vi "_Engine.vi"(6 "Enum":T1, 7 "Module Name":string, 8 "Error in":errorcluster caption="Error in (no error)", 11 "Message":string) -> (0 "Error out":errorcluster, 2 "Array":string[](array[string]), 3 "Message Event":refnum<user-event>)   [LabVIEW 2017, in "_csmlite.lvlib"]
uses:
  _csmlite.lvlib
  _action.ctl
  _Shared/CSM Shared.lvlib
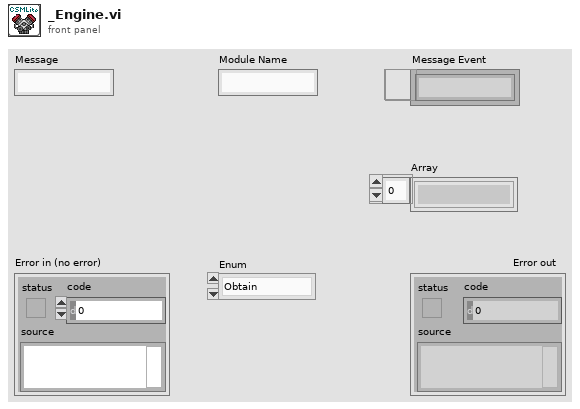
[diagram p1: front panel]
types:
  T1 = typedef "_csmlite.lvlib/_action.ctl" = enum16{"Obtain", "Destroy", "Broadcast", "Post", "List"}
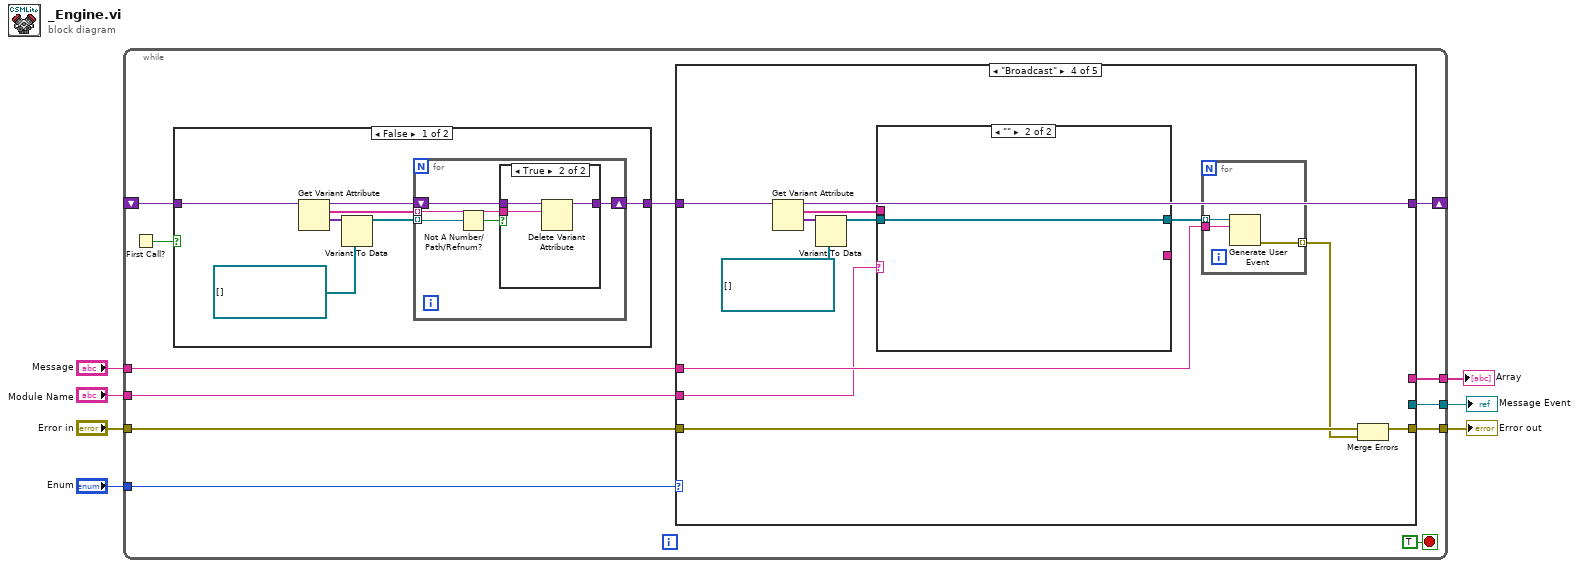
[diagram p0: block diagram]
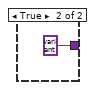
[diagram p3: hidden frame]
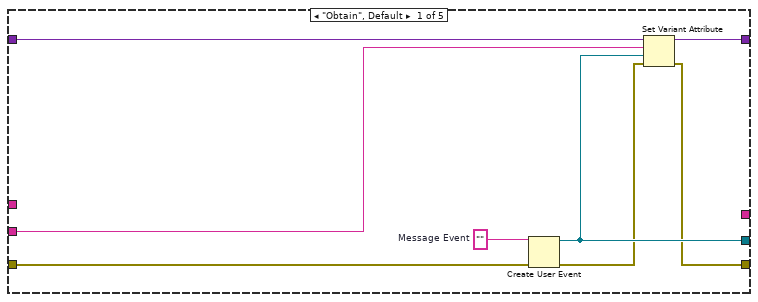
[diagram p4: hidden frame]
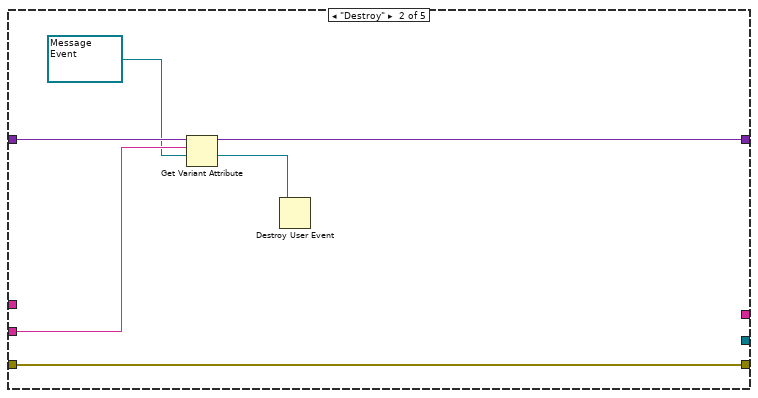
[diagram p5: hidden frame]
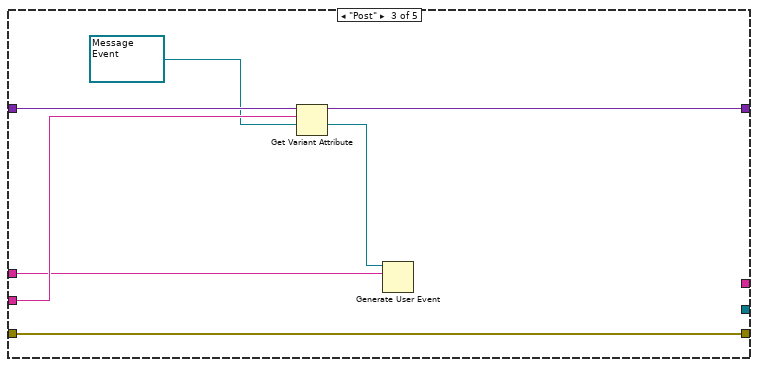
[diagram p6: hidden frame]
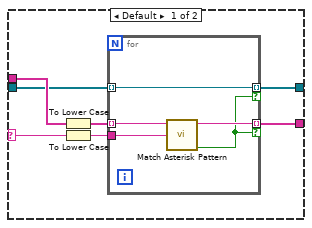
[diagram p7: hidden frame]
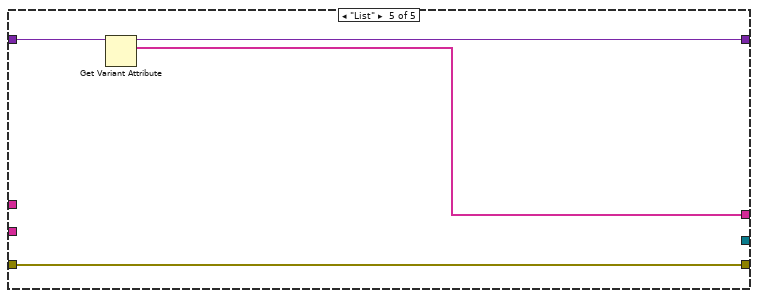
[diagram p8: hidden frame]
diagram:
  n1 = while {
    tunnel: [w18] -> w7
    tunnel: [w17] -> w6
    tunnel: "Error in" -> [w16]
    tunnel: "Enum" -> [w15]
    shift-right: [w14] -> _
    shift-left: _ -> [w12]
    tunnel: "Module Name" -> [w10]
    tunnel: "Message" -> [w9]
    tunnel: [w8] -> w1
    stop <- TRUE stop-if-true
    n2 = First Call?() -> (First Call?: T/F=w11:bool)
    n3 = case shown="False" w11 {
      tunnel: [w25 variant] -> w13
      tunnel: w12 -> [w26 _]
      frame False {
        n4 = Get Variant Attribute(Variant=w26) -> (duplicate Variant=w24:variant, names=w23:string[], values=w22:variant[])  [unwired: 3 in, 1 out]
        n5 = Variant To Data(type=refnum<user-event>[] [], Variant=w22) -> (data=w20:refnum<user-event>[])  [unwired: 1 in, 1 out]
        n6 = for {
          shift-right: [w30] -> w25
          shift-left: w24 -> [w31]
          tunnel: w23 -> [w29] mode=indexing
          tunnel: w20 -> [w28] mode=indexing
          n7 = Not A Number/Path/Refnum?(number/path/refnum=w28) -> (NaN/Path/Refnum?=w27:bool)
          n8 = case shown="True" w27 {
            tunnel: w31 -> [w32 w35]
            tunnel: [w32 w34] -> w30
            tunnel: w29 -> [_ w33]
            frame False {
            }
            frame True {
              n9 = Delete Variant Attribute(6:w33, 7:w35) -> (3:w34:variant)  [unwired: 1 in, 2 out]
            }
          }
        }
      }
      frame True {
      }
    }
    n10 = case shown="\"Broadcast\"" w15 {
      tunnel: [w39 _ _ _ _] -> w18
      tunnel: [w37 w49 w56 w63 w89] -> w17
      tunnel: w16 -> [w43 w49 w56 w69 w89]
      tunnel: [w41 w48 w55 w65 w87] -> w14
      tunnel: w13 -> [w42 w50 w57 w66 w88]
      tunnel: w10 -> [w40 w47 w54 w61 _]
      tunnel: w9 -> [_ _ w52 w64 _]
      tunnel: [_ _ _ _ w86] -> w8
      frame "Obtain", Default {
        w44 = ""  # Message Event
        n11 = Create User Event(user event datatype=w44, error in=w43) -> (user event=w39:refnum<user-event>, error out=w38:errorcluster)
        n12 = Set Variant Attribute(Variant=w42, name=w40, value=w39, error in=w38) -> (Variant out=w41:variant, error out=w37:errorcluster)  [unwired: 1 out]
      }
      frame "Destroy" {
        n13 = Get Variant Attribute(Variant=w50, name=w47, default value (empty Variant)=refnum<user-event> refnum ("CSMLite")) -> (duplicate Variant=w48:variant, value=w46:refnum<user-event>)  [unwired: 1 in, 2 out]
        n14 = Destroy User Event(user event=w46) -> ()  [unwired: 1 in, 1 out]
      }
      frame "Post" {
        n15 = Get Variant Attribute(Variant=w57, name=w54, default value (empty Variant)=refnum<user-event> refnum ("CSMLite")) -> (duplicate Variant=w55:variant, value=w53:refnum<user-event>)  [unwired: 1 in, 2 out]
        n16 = Generate User Event(user event=w53, event data cluster=w52) -> ()  [unwired: 2 in, 2 out]
      }
      frame "Broadcast" {
        n17 = Get Variant Attribute(Variant=w66) -> (duplicate Variant=w65:variant, names=w60:string[], values=w67:variant[])  [unwired: 3 in, 1 out]
        n18 = Variant To Data(type=refnum<user-event>[] [], Variant=w67) -> (data=w59:refnum<user-event>[])  [unwired: 1 in, 1 out]
        n19 = case shown="\"\"" w61 {
          selector: w61 -> [w75 _]
          tunnel: w60 -> [w76 _]
          tunnel: w59 -> [w73 w82]
          tunnel: [w74 w82] -> w58
          tunnel: [w72 _] -> _
          frame Default {
            n20 = To Lower Case(string=w76) -> (all lower case string=w71:string[])
            n21 = To Lower Case(string=w75) -> (all lower case string=w70:string)
            n22 = for {
              tunnel: w71 -> [w81] mode=indexing
              tunnel: w70 -> [w80]
              tunnel: [w79] -> w74 mode=indexing if=w77
              tunnel: w73 -> [w79] mode=indexing
              tunnel: [w78] -> w72 mode=indexing if=w77
              n23 = call "Match Asterisk Pattern.vi"("String"=w81, "* Expression"=w80) -> ("String (Dup)"=w78:string, "Matched"=w77:bool)  [unwired: 7 in]
            }
          }
          frame "" {
          }
        }
        n24 = for {
          tunnel: w58 -> [w85] mode=indexing
          tunnel: w64 -> [w84]
          tunnel: [w83] -> w62 mode=indexing
          n25 = Generate User Event(user event=w85, event data cluster=w84) -> (error out=w83:errorcluster)  [unwired: 2 in, 1 out]
        }
        n26 = Merge Errors(w69, w62) -> (w63:errorcluster)
      }
      frame "List" {
        n27 = Get Variant Attribute(Variant=w88) -> (duplicate Variant=w87:variant, names=w86:string[])  [unwired: 3 in, 2 out]
      }
    }
  }
  "Error out" <- w6
  "Message Event" <- w7
  "Array" <- w1
